vi "Get Scanner Fine.vi"(8 "error in (no error)":errorcluster, 11 "Translation Stages in":refnum<class "Translation Stages.lvclass">) -> (0 "error out":errorcluster, 2 "Default Scanner out":refnum<class "Scanner.lvclass">)   [LabVIEW 2015, in "Translation Stages.lvclass"]
uses:
  Translation Stages.lvclass
  Scanners/Scanner/Scanner.lvclass
  Scanners/Translation Stage Fine/Translation Stage Fine.lvclass
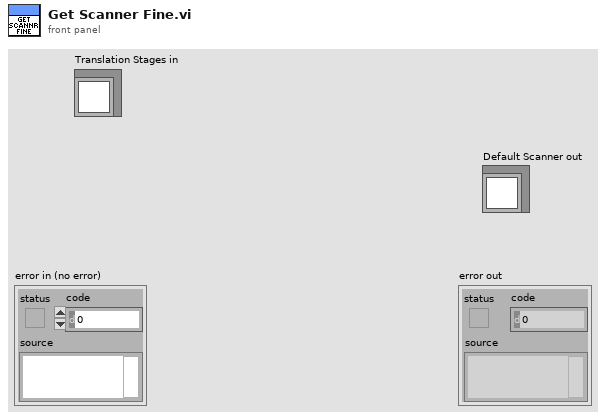
[diagram p1: front panel]
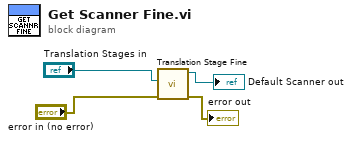
[diagram p0: block diagram]
diagram:
  n1 = call "Translation Stage Fine.vi"("error in (no error)"="error in (no error)", "Translation Stages.lvclass"="Translation Stages in") -> ("error out"=→"error out":errorcluster, "Translation Stage Fine Out"=→"Default Scanner out":refnum<class "Translation Stage Fine.lvclass">)  [unwired: 8 in]
